vi "RT Main.vi"   [LabVIEW 2020]
doc: "This template is for the Queued Message Handler design pattern.\n\nThe Event Handling Loop generates messages based on user interface actions.\n\nThe Message Handling Loop processes messages generated by the Event Handling Loop, or by other messages. The messages are string values, so new messages can be added easily to the Message Cases case structure in the Message Handling Loop. Each message cluster can also provide an optional value for Message Data, which is a variant that can be converted to whatever message-specific data is required."
uses:
  Globals/Global - All RT Loop Stop.vi
  Globals/Global - Monitoring Variables.vi
  Globals/Global - Configuration Options.vi
  Globals/Global - RT Stream Connections.vi
  support/Message Queue/Message Queue.lvlib
  <vilib>/nisyscfg/nisyscfg.lvlib
types:
  T1 = typedef "Acquisition and Logging Configuration.ctl" = cluster{"Data Rate":T2, "Samples per Read":i32, "Number of Reads to Save":i32, "Data File Name":string, "TDMS Properties":T3[], "Number of Channels":i32, "Channel Scale Array":fxp<+,24,12>[], "Channel Names":string[], "Trigger - RMS Value":dbl, "Trigger - Channel":i32, "Trigger - Time (Minute)":i32}
  T2 = typedef "nicrio_cRIO-9234_DataRatesRing2.ctl" = u8
  T3 = typedef "TDMS Properties.ctl" = cluster{"Name":string, "Value":string}
  T4 = typedef "Message Queue.lvlib/All Real-Time Message Queues.ctl" = cluster{"Message Handler":refnum<queue>, "Acquisition and Logging":refnum<queue>, "Actuation":refnum<queue>}
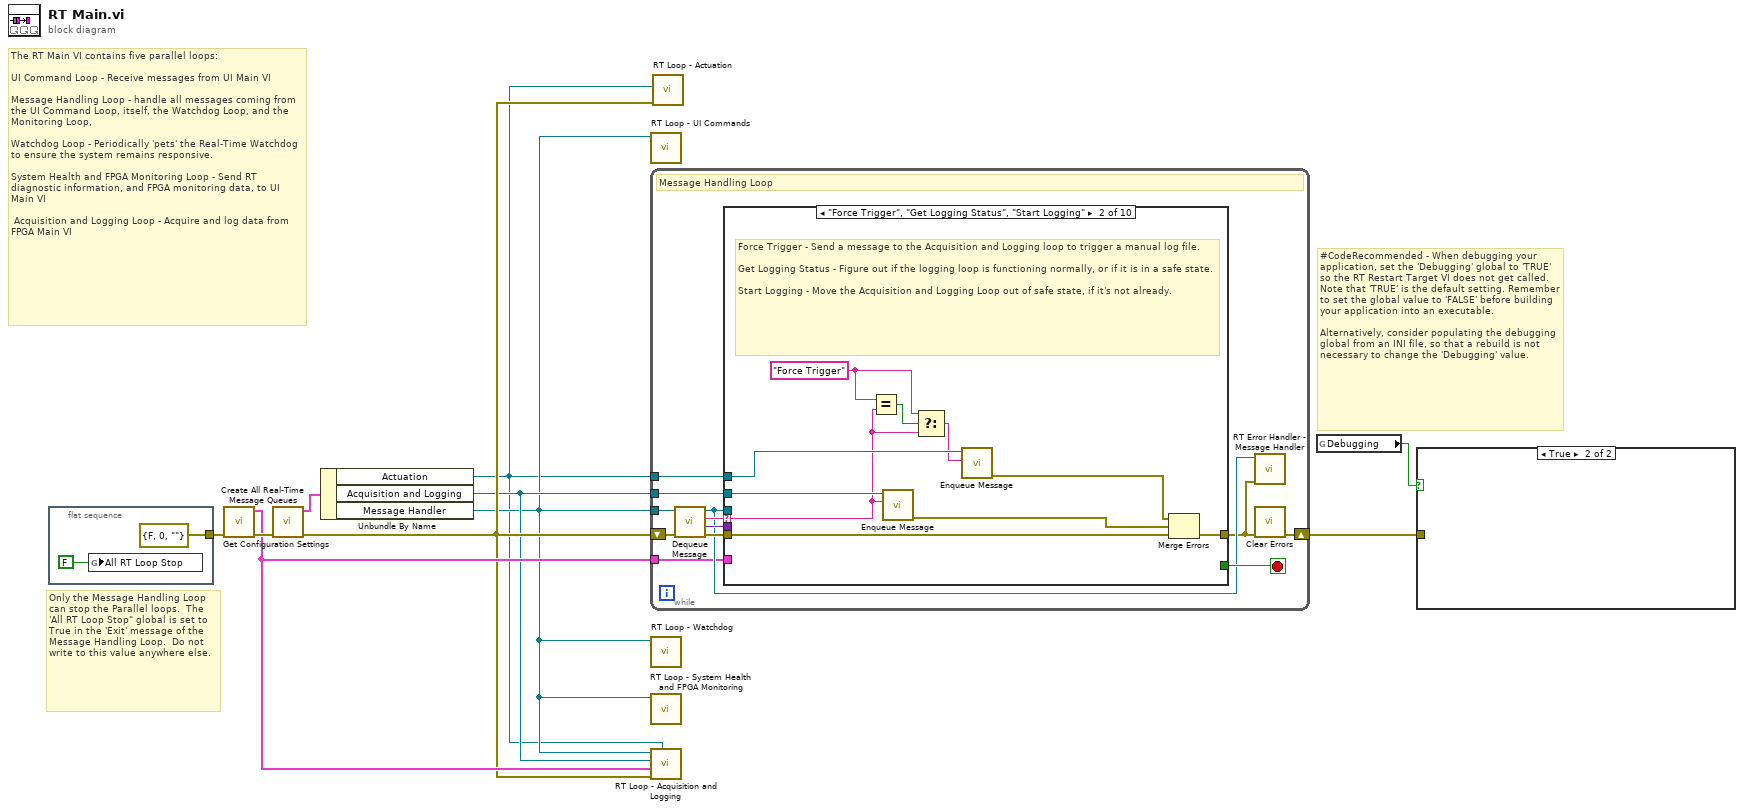
[diagram p0: block diagram]
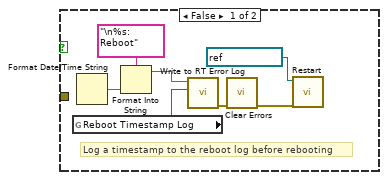
[diagram p2: hidden frame]
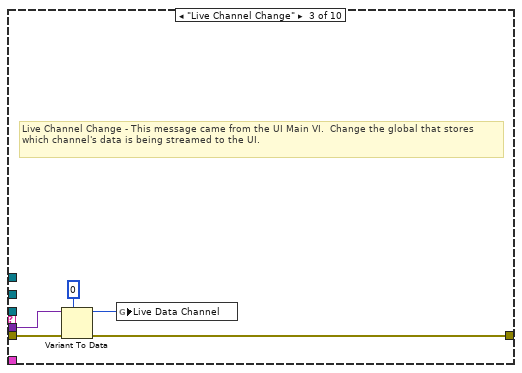
[diagram p4: hidden frame]
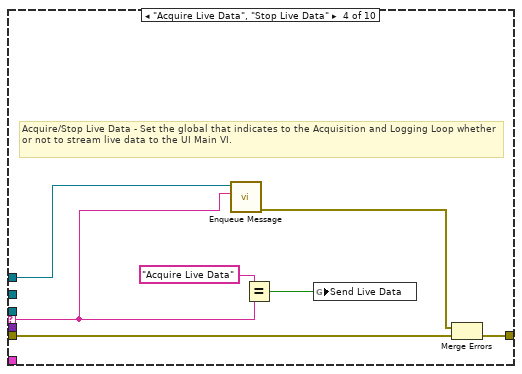
[diagram p5: hidden frame]
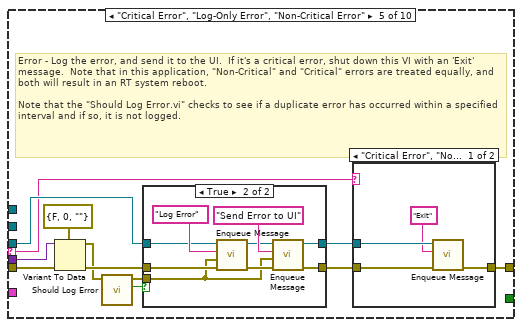
[diagram p6: hidden frame]
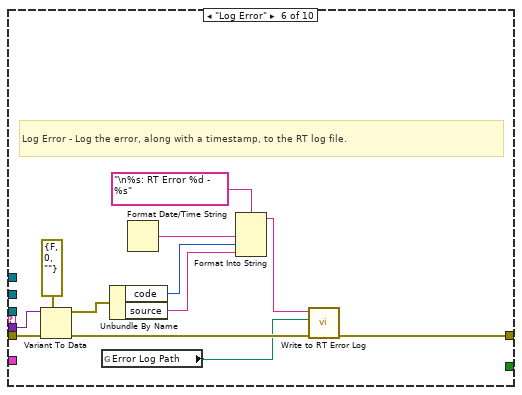
[diagram p9: hidden frame]
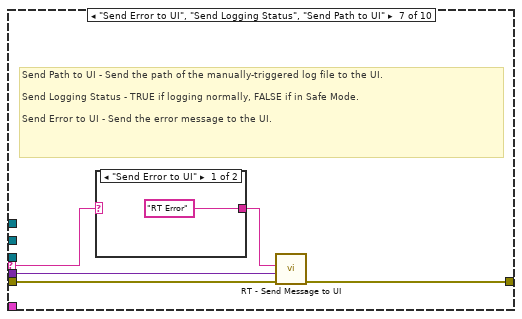
[diagram p10: hidden frame]
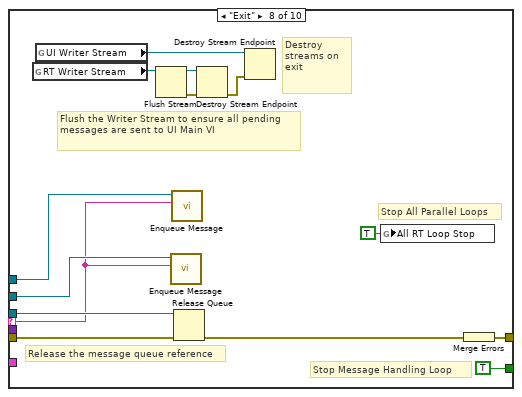
[diagram p12: hidden frame]
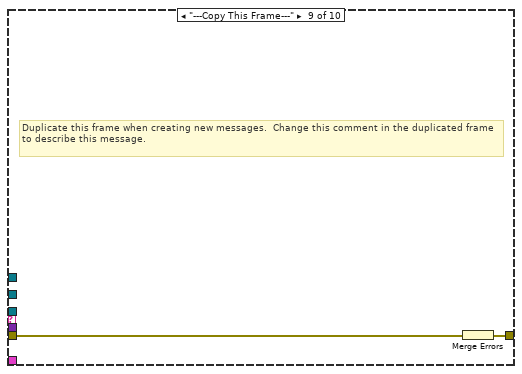
[diagram p13: hidden frame]
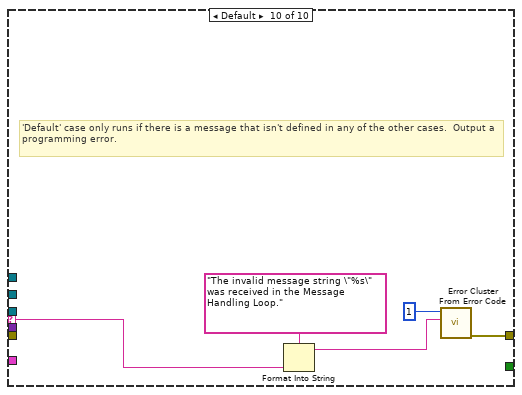
[diagram p14: hidden frame]
diagram:
  # "#CodeRecommended - When debugging your application, set the 'Debugging' global to 'TRUE' so the RT Restart Target VI does not get called.  Note that 'TRUE' is the default setting. Remember to set the global value to 'FALSE' before building your application into an executable.\n\nAlternatively, consider populating the debugging global from an INI file, so that a rebuild is not necessary to change the 'Debugging' value."
  # "The RT Main VI contains five parallel loops:\n\nUI Command Loop - Receive messages from UI Main VI\n\nMessage Handling Loop - handle all messages coming from the UI Command Loop, itself, the Watchdog Loop, and the Monitoring Loop, \n\nWatchdog Loop - Periodically 'pets' the Real-Time Watchdog to ensure the system remains responsive.\n\nSystem Health and FPGA Monitoring Loop - Send RT diagnostic information, and FPGA monitoring data, to UI Main VI\n\n Acquisition and Logging Loop - Acquire and log data from FPGA Main VI"
  # "Only the Message Handling Loop can stop the Parallel loops.  The 'All RT Loop Stop\" global is set to True in the 'Exit' message of the Message Handling Loop.  Do not write to this value anywhere else."
  n1 = flat-sequence {
    tunnel: [errorcluster {"status"=FALSE, "code"=0, "source"=""} ("error constant")] -> w10
    frame #0 {
      n2 = global write "Global - All RT Loop Stop.vi" "All RT Loop Stop"(FALSE) -> ()
    }
  }
  n3 = call "Get Configuration Settings.vi"("error in (no error)"=w10) -> ("error out"=w7:errorcluster, "Acquisition and Logging Configuration"=w5:T1)  [unwired: 9 in]
  n4 = call "Create All Real-Time Message Queues.vi"("error in (no error)"=w7) -> ("error out"=w4:errorcluster, "Message Queues out"=w6:T4)  [unwired: 9 in]
  n5 = Unbundle By Name(w6) -> ("Actuation"=w1:refnum<queue>, "Acquisition and Logging"=w3:refnum<queue>, "Message Handler"=w2:refnum<queue>)
  n6 = call "RT Loop - UI Commands.vi"("Message Queue"=w2) -> ()  [unwired: 11 in]
  n7 = while {
    tunnel: w2 -> [w19]
    shift-right: [w17] -> w9
    shift-left: w4 -> [w23]
    tunnel: w3 -> [w15]
    tunnel: w5 -> [w14]
    tunnel: w1 -> [w13]
    stop <- w24 stop-if-true
    # "Message Handling Loop"
    n8 = call "Dequeue Message.vi"("error in (no error)"=w23, "Message Queue"=w19) -> ("error out"=w22:errorcluster, "Message Data"=w20:variant, "Message"=w21:string, "dup Message Queue"=w18:refnum<queue>)  [unwired: 6 in]
    n9 = case "Message Cases" shown="\"Force Trigger\", \"Get Logging Status\", \"Start Logging\"" w21 {
      selector: w21 -> [_ w26 _ w45 w53 _ w89 w95 _ w114]
      tunnel: w18 -> [_ _ _ _ w54 _ _ w108 _ _]
      tunnel: w22 -> [w25 w35 w40 w42 w56 w87 w92 w104 w110 _]
      tunnel: [w25 w33 w39 w43 w59 w78 w91 w105 w109 w112] -> w16
      tunnel: [_ _ _ _ _ _ _ TRUE _ _] -> w24
      tunnel: w20 -> [_ _ w38 _ w48 w86 w90 _ _ _]
      tunnel: w15 -> [_ w34 _ _ _ _ _ w99 _ _]
      tunnel: w14 -> [_ _ _ _ _ _ _ _ _ _]
      tunnel: w13 -> [_ w31 _ w44 _ _ _ w96 _ _]
      frame "Initialize" {
        # "Initialize - Currently a no-op for the RT Main VI"
      }
      frame "Force Trigger", "Get Logging Status", "Start Logging" {
        w28 = "Force Trigger" ("x")
        # "Force Trigger - Send a message to the Acquisition and Logging loop to trigger a manual log file.\n\nGet Logging Status - Figure out if the logging loop is functioning normally, or if it is in a safe state.\n\nStart Logging - Move the Acquisition and Logging Loop out of safe state, if it's not already."
        n10 = Equal?(x=w28, y=w26) -> (x = y?=w27:bool)
        n11 = call "Enqueue Message.vi"("Message"=w26, "Message Queue"=w34) -> ("error out"=w32:errorcluster)  [unwired: 8 in, 1 out]
        n12 = Select(t=w28, s=w27, f=w26) -> (s? t:f=w29:string)
        n13 = call "Enqueue Message.vi"("Message"=w29, "Message Queue"=w31) -> ("error out"=w30:errorcluster)  [unwired: 8 in, 1 out]
        n14 = Merge Errors(w30, w32, w35) -> (w33:errorcluster)
      }
      frame "Live Channel Change" {
        # "Live Channel Change - This message came from the UI Main VI.  Change the global that stores which channel's data is being streamed to the UI."
        n15 = Variant To Data(error in=w40, type=u32 0, Variant=w38) -> (data=w36:u32, error out=w39:errorcluster)
        n16 = global write "Global - Monitoring Variables.vi" "Live Data Channel"(w36) -> ()
      }
      frame "Acquire Live Data", "Stop Live Data" {
        # "Acquire/Stop Live Data - Set the global that indicates to the Acquisition and Logging Loop whether or not to stream live data to the UI Main VI."
        n17 = call "Enqueue Message.vi"("Message"=w45, "Message Queue"=w44) -> ("error out"=w41:errorcluster)  [unwired: 8 in, 1 out]
        n18 = Equal?(x="Acquire Live Data", y=w45) -> (x = y?=w46:bool)
        n19 = global write "Global - Monitoring Variables.vi" "Send Live Data"(w46) -> ()
        n20 = Merge Errors(w41, w42) -> (w43:errorcluster)
      }
      frame "Critical Error", "Log-Only Error", "Non-Critical Error" {
        # "Error - Log the error, and send it to the UI.  If it's a critical error, shut down this VI with an 'Exit' message.  Note that in this application, \"Non-Critical\" and \"Critical\" errors are treated equally, and both will result in an RT system reboot.\n\nNote that the \"Should Log Error.vi\" checks to see if a duplicate error has occurred within a specified interval and if so, it is not logged."
        n21 = Variant To Data(error in=w56, type=errorcluster {"status"=FALSE, "code"=0, "source"=""} ("error out"), Variant=w48) -> (data=w51:errorcluster, error out=w57:errorcluster)
        n22 = call "Should Log Error.vi"("error to report"=w51) -> ("Should Log Error?"=w49:bool, "dup error to report"=w50:errorcluster)  [unwired: 9 in]
        n23 = case shown="True" w49 {
          tunnel: [w61 w68] -> w55
          tunnel: [w60 w67] -> w52
          tunnel: w54 -> [w60 w66]
          tunnel: w57 -> [w61 w63]
          tunnel: w50 -> [_ w62]
          frame False {
          }
          frame True {
            n24 = call "Enqueue Message.vi"("error in (no error)"=w63, "Message Data"=w62, "Message"="Log Error", "Message Queue"=w66) -> ("error out"=w64:errorcluster, "dup Message Queue"=w65:refnum<queue>)  [unwired: 6 in]
            n25 = call "Enqueue Message.vi"("error in (no error)"=w64, "Message Data"=w62, "Message"="Send Error to UI", "Message Queue"=w65) -> ("error out"=w68:errorcluster, "dup Message Queue"=w67:refnum<queue>)  [unwired: 6 in]
          }
        }
        n26 = case shown="\"Critical Error\", \"Non-Critical Error\"" w53 {
          tunnel: w55 -> [w74 w75]
          tunnel: w52 -> [w72 _]
          tunnel: [w73 w75] -> w59
          frame "Critical Error", "Non-Critical Error" {
            n27 = call "Enqueue Message.vi"("error in (no error)"=w74, "Message"="Exit", "Message Queue"=w72) -> ("error out"=w73:errorcluster)  [unwired: 7 in, 1 out]
          }
          frame Default {
          }
        }
      }
      frame "Log Error" {
        # "Log Error - Log the error, along with a timestamp, to the RT log file."
        n28 = Variant To Data(error in=w87, type=errorcluster {"status"=FALSE, "code"=0, "source"=""} ("error constant"), Variant=w86) -> (data=w81:errorcluster, error out=w84:errorcluster)
        n29 = global read "Global - Configuration Options.vi" "Error Log Path"() -> (w76:path)
        n30 = Unbundle By Name(w81) -> ("code"=w80:i32, "source"=w79:string)
        n31 = Format Date/Time String() -> (date/time string=w82:string)  [unwired: 3 in]
        n32 = Format Into String(format string="\n%s: RT Error %d - %s", w82, w80, w79) -> (resulting string=w77:string)  [unwired: 2 in, 1 out]
        n33 = call "Write to RT Error Log.vi"("error in (no error)"=w84, "Error Log Path"=w76, "Log Entry"=w77) -> ("error out"=w78:errorcluster)  [unwired: 8 in]
      }
      frame "Send Error to UI", "Send Logging Status", "Send Path to UI" {
        # "Send Path to UI - Send the path of the manually-triggered log file to the UI.\n\nSend Logging Status - TRUE if logging normally, FALSE if in Safe Mode.\n\nSend Error to UI - Send the error message to the UI."
        n34 = case shown="\"Send Error to UI\"" w89 {
          selector: w89 -> [_ w94]
          tunnel: ["RT Error" ("Message") w94] -> w88
          frame "Send Error to UI" {
          }
          frame Default {
          }
        }
        n35 = call "RT - Send Message to UI.vi"("error in (no error)"=w92, "Message Data"=w90, "Message"=w88) -> ("error out"=w91:errorcluster)  [unwired: 8 in]
      }
      frame "Exit" {
        # "Flush the Writer Stream to ensure all pending messages are sent to UI Main VI"
        # "Destroy streams on exit"
        # "Stop Message Handling Loop"
        # "Stop All Parallel Loops"
        # "Release the message queue reference"
        n36 = global read "Global - RT Stream Connections.vi" "RT Writer Stream"() -> (w102:refnum<k21>)
        n37 = global read "Global - RT Stream Connections.vi" "UI Writer Stream"() -> (w101:refnum<k21>)
        n38 = Flush Stream(11:w102) -> (0:w97:errorcluster, 3:w98:refnum<k21>)  [unwired: 3 in, 1 out]
        n39 = call "Enqueue Message.vi"("Message"=w95, "Message Queue"=w99) -> ()  [unwired: 8 in, 2 out]
        n40 = call "Enqueue Message.vi"("Message"=w95, "Message Queue"=w96) -> ()  [unwired: 8 in, 2 out]
        n41 = Release Queue(queue=w108, error in (no error)=w104) -> (error out=w106:errorcluster)  [unwired: 1 in, 2 out]
        n42 = Destroy Stream Endpoint(8:w97, 11:w98) -> (0:w100:errorcluster)
        n43 = Destroy Stream Endpoint(8:w100, 11:w101) -> ()  [unwired: 1 out]
        n44 = global write "Global - All RT Loop Stop.vi" "All RT Loop Stop"(TRUE ("Stop Monitoring Loops")) -> ()
        n45 = Merge Errors(w106) -> (w105:errorcluster)
      }
      frame "---Copy This Frame---" {
        # "Duplicate this frame when creating new messages.  Change this comment in the duplicated frame to describe this message."
        n46 = Merge Errors(w110) -> (w109:errorcluster)
      }
      frame Default {
        # "'Default' case only runs if there is a message that isn't defined in any of the other cases.  Output a programming error."
        n47 = Format Into String(format string="The invalid message string \"%s\" was received in the Message Handling Loop." ("Unknown Message Error Text"), w114) -> (resulting string=w111:string)  [unwired: 2 in, 1 out]
        n48 = call <vilib>:"Error Cluster From Error Code.vi"("error message (\"\")"=w111, "error code (0)"=1) -> ("error out"=w112:errorcluster)  [unwired: 7 in]
      }
    }
    n49 = call "RT Error Handler - Message Handler.vi"("error in (no error)"=w16, "Message Queue"=w18) -> ()  [unwired: 9 in, 1 out]
    n50 = call <vilib>:"Clear Errors.vi"("error in (no error)"=w16) -> ("error out"=w17:errorcluster)  [unwired: 5 in, 1 out]
  }
  n51 = call "RT Loop - Watchdog.vi"("Message Queue"=w2) -> ()  [unwired: 11 in]
  n52 = call "RT Loop - System Health and FPGA Monitoring.vi"("Message Queue"=w2) -> ()  [unwired: 11 in]
  n53 = call "RT Loop - Acquisition and Logging.vi"("Actuation Queue"=w1, "error in (no error)"=w4, "Acquisition and Logging Configuration"=w5, "Acquisition and Logging Queue"=w3, "Message Queue"=w2) -> ()  [unwired: 7 in]
  n54 = call "RT Loop - Actuation.vi"("error in (no error)"=w4, "Actuation Queue"=w1) -> ()  [unwired: 10 in]
  n55 = global read "Global - Configuration Options.vi" "Debugging"() -> (w8:bool)
  n56 = case shown="True" w8 {
    tunnel: w9 -> [_ _]
    frame False {
      # "Log a timestamp to the reboot log before rebooting"
      n57 = global read "Global - Configuration Options.vi" "Reboot Timestamp Log"() -> (w118:path)
      n58 = Format Date/Time String() -> (date/time string=w120:string)  [unwired: 3 in]
      n59 = Format Into String(format string="\n%s: Reboot", w120) -> (resulting string=w119:string)  [unwired: 2 in, 1 out]
      n60 = call "Write to RT Error Log.vi"("Error Log Path"=w118, "Log Entry"=w119) -> ("error out"=w122:errorcluster)  [unwired: 9 in]
      n61 = call <vilib>:"Clear Errors.vi"("error in (no error)"=w122) -> ("error out"=w117:errorcluster)  [unwired: 5 in, 1 out]
      n62 = call <vilib>:"Restart.vi"("error in (no error)"=w117, "Session in"=refnum<k21> "localhost" ("session in")) -> ()  [unwired: 7 in, 3 out]
    }
    frame True {
    }
  }
